vi "next stmt.vi"(8 "error in (no error)":errorcluster, 10 "pStmt":dbl, 11 "pDb":dbl) -> (0 "error out":errorcluster, 1 "function return":u32, 2 "pStmt out":dbl, 3 "pDb out":dbl)   [LabVIEW 2020, in "sqlite3.lvlib"]
uses:
  sqlite3.lvlib
  errstr.vi
  bin/sqlite3_64.dll
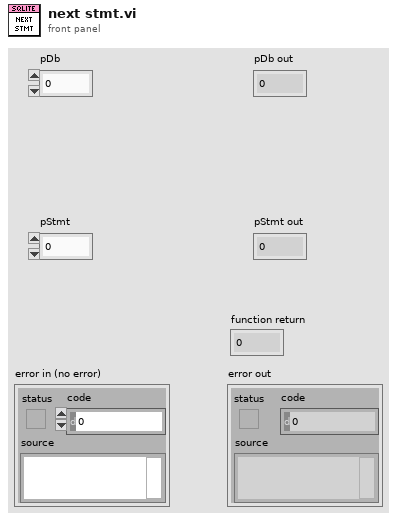
[diagram p1: front panel]
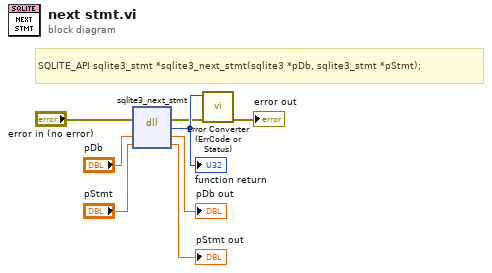
[diagram p0: block diagram]
diagram:
  # "SQLITE_API sqlite3_stmt *sqlite3_next_stmt(sqlite3 *pDb, sqlite3_stmt *pStmt);"
  n1 = dll-call lib="D:/Project/Labview-Projects/database-configuration/externals/sqlite3/Source/bin/sqlite3_*.*" fn="sqlite3_next_stmt"(error in="error in (no error)", "pDb"="pDb", "pStmt"="pStmt") -> (error out=w2:errorcluster, w8:u32, "pDb"=→"pDb out":dbl, "pStmt"=→"pStmt out":dbl)  [unwired: 2 in, 1 out]
  "function return" <- w8
  n2 = call "Error Converter (ErrCode or Status).vi"("error in (no error)"=w2, "error code"=w8) -> ("error out"=→"error out":errorcluster)  [unwired: 9 in]
